vi "ComputerRemote.vi"() -> ()   [LabVIEW 2020]
uses:
  LMH-PS4/Private/Type Defs/Indicators/Controller.ctl
  LMH-PS4/Private/Type Defs/Indicators/Square.ctl
  LMH-PS4/Private/Type Defs/Indicators/X.ctl
  LMH-PS4/Private/Type Defs/Indicators/Circle.ctl
  LMH-PS4/Private/Type Defs/Indicators/Triangle.ctl
  LMH-PS4/Private/Type Defs/Indicators/L1.ctl
  LMH-PS4/Private/Type Defs/Indicators/R1.ctl
  LMH-PS4/Private/Type Defs/Indicators/Share.ctl
  LMH-PS4/Private/Type Defs/Indicators/Options.ctl
  LMH-PS4/Private/Type Defs/Indicators/PS.ctl
  LMH-PS4/Private/Type Defs/Indicators/Pad_Button.ctl
  LMH-PS4/Private/Type Defs/Indicators/Dpad.ctl
  LMH-PS4/Private/Type Defs/Indicators/Slider.ctl
  LMH-PS4/Public/Open First Controller.vi
  LMH-PS4/LMH-PS4.lvlib
  <vilib>/ReMiSYS Technology/RemoteToolkit/Sender/Sender.lvclass
panel:
  out "D-Pad":T1=5
  out "R2":T2 scale=-32768.0..32767.0
  out "L2":T2 scale=-32768.0..32767.0
  in  "IP Address":string="10.12.34.2"
  in  "Stop Button":bool
  out "PS4 Controller":T3={"Square Button"=FALSE, "X Button"=FALSE, "Circle Button"=FALSE, "Triangle Button"=FALSE, "L1"=FALSE, "R1"=FALSE, "Share Button"=FALSE, "Options Button"=FALSE, "PS Button"=FALSE, "Pad Button"=FALSE, "D-Pad"=5, "L2"=0, "R2"=0, "Thumbstick_Left"={[], []}, "Thumbstick_Right"={[], []}} {"R2" scale=-32768.0..32767.0; "L2" scale=-32768.0..32767.0}
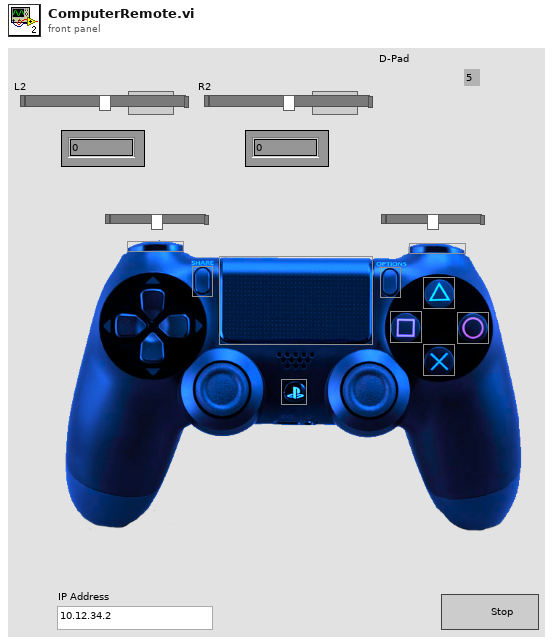
[diagram p1: front panel]
types:
  T1 = typedef "LMH-PS4.lvlib/Dpad.ctl" = u16
  T2 = typedef "LMH-PS4.lvlib/Slider.ctl" = i32
  T3 = typedef "LMH-PS4.lvlib/Controller.ctl" = cluster{"Square Button":T4, "X Button":T5, "Circle Button":T6, "Triangle Button":T7, "L1":T8, "R1":T9, "Share Button":T10, "Options Button":T11, "PS Button":T12, "Pad Button":T13, "D-Pad":T1, "L2":T2, "R2":T2, "Thumbstick_Left":cluster{i32[], i32[]}, "Thumbstick_Right":cluster{i32[], i32[]}}
  T4 = typedef "LMH-PS4.lvlib/Square.ctl" = bool
  T5 = typedef "LMH-PS4.lvlib/X.ctl" = bool
  T6 = typedef "LMH-PS4.lvlib/Circle.ctl" = bool
  T7 = typedef "LMH-PS4.lvlib/Triangle.ctl" = bool
  T8 = typedef "LMH-PS4.lvlib/L1.ctl" = bool
  T9 = typedef "LMH-PS4.lvlib/R1.ctl" = bool
  T10 = typedef "LMH-PS4.lvlib/Share.ctl" = bool
  T11 = typedef "LMH-PS4.lvlib/Options.ctl" = bool
  T12 = typedef "LMH-PS4.lvlib/PS.ctl" = bool
  T13 = typedef "LMH-PS4.lvlib/Pad_Button.ctl" = bool
  T14 = typedef "LMH-PS4.lvlib/PS4 Controller Ref.ctl" = cluster{"Controller Ref":refnum<k1>, "PS4 Events Ref":refnum<event-registration>, "Worker Ref":refnum<vi>}
  T15 = typedef "LMH-PS4.lvlib/Axis.ctl" = cluster{"Left Thumbstick":cluster{"X Axis":i32, "Y Axis":i32}, "Right Thumbstick":cluster{"X Axis":i32, "Y Axis":i32}, "L2":i32, "R2":i32, "D-Pad":T16}
  T16 = typedef "LMH-PS4.lvlib/DPad Enum.ctl" = enum16{"Idle", "Up", "Up / Right", "Right", "Down / Right", "Down", "Down / Left", "Left", "Up / Left"}
  T17 = typedef "LMH-PS4.lvlib/Buttons.ctl" = cluster{"Square":bool, "X":bool, "Circle":bool, "Triangle":bool, "L1":bool, "R1":bool, "L2":bool, "R2":bool, "Share":bool, "Options":bool, "Left Thumbstick":bool, "Right Thumbstick":bool, "Playstation Button":bool, "Pad":bool}
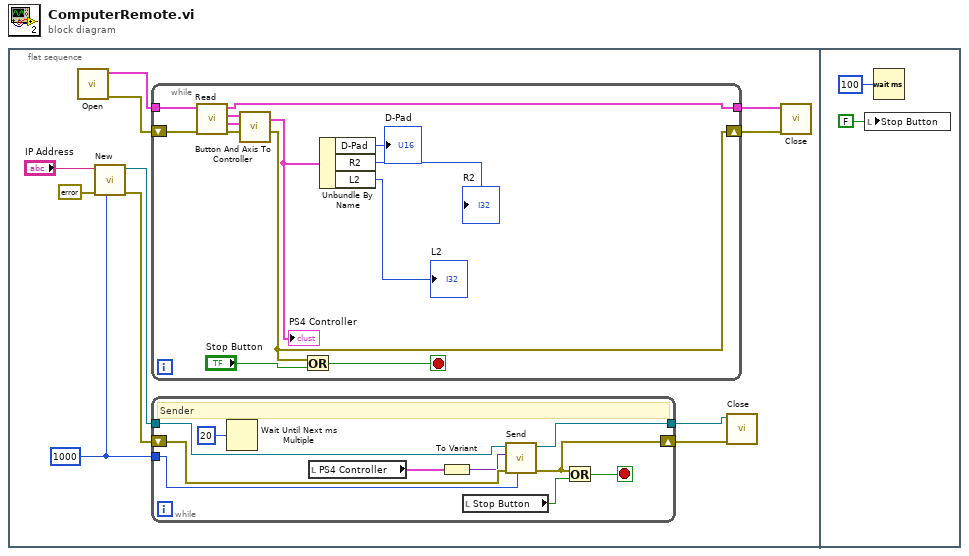
[diagram p0: block diagram]
diagram:
  n1 = flat-sequence {
    frame #0 {
      w5 = 1000 ("Timeout ms (25000)")
      n2 = call-poly "Open.vi"() -> ("Error Out"=w9:errorcluster, "PS4 Controller Ref"=w8:T14)  [unwired: 9 in, 1 out]
      n3 = call <vilib>:"New.vi"("Timeout ms (25000)"=w5, "Error In"=errorcluster {"status"=FALSE, "code"=0, "source"=""}, "IP Address"="IP Address") -> ("Error Out"=w6:errorcluster, "Sender Ref."=w3:refnum<class "Sender.lvclass">)  [unwired: 7 in]
      n4 = while {
        shift-right: [w29] -> w11
        shift-left: w9 -> [w26]
        tunnel: [w28] -> w10
        tunnel: w8 -> [w27]
        stop <- w31 stop-if-true
        n5 = call "Read.vi"("Error In"=w26, "PS4 Controller Ref"=w27) -> ("Error Out"=w29:errorcluster, "All Axis"=w33:T15, "Buttons"=w32:T17, "PS4 Controller Ref"=w28:T14)  [unwired: 6 in]
        n6 = call "Button And Axis To Controller.vi"("All Axis"=w33, "Buttons"=w32) -> ("PS4 Controller"=w25:T3)  [unwired: 5 in]
        "PS4 Controller" <- w25
        n7 = Or(x=w29, y="Stop Button") -> (x .or. y?=w31:bool)
        n8 = Unbundle By Name(w25) -> ("D-Pad"=→"D-Pad":T1, "R2"=→"R2":T2, "L2"=→"L2":T2)
      }
      n9 = while {
        shift-right: [w17] -> w2
        shift-left: w6 -> [w19]
        tunnel: w3 -> [w20]
        tunnel: w5 -> [w15]
        tunnel: [w18] -> w1
        stop <- w21 stop-if-true
        # "Sender"
        n10 = Wait Until Next ms Multiple(millisecond multiple=u32 20) -> ()  [unwired: 1 out]
        n11 = local read "PS4 Controller"() -> (w13:T3)
        n12 = To Variant(anything=w13) -> (Variant=w16:variant)
        n13 = local read "Stop Button"() -> (w12:bool)
        n14 = call <vilib>:"Send.vi"("Timeout ms (1000)"=w15, "Error In"=w19, "Value"=w16, "Sender Ref."=w20) -> ("Error Out"=w17:errorcluster, "Sender Ref."=w18:refnum<class "Sender.lvclass">)  [unwired: 6 in]
        n15 = Or(x=w17, y=w12) -> (x .or. y?=w21:bool)
      }
      n16 = call <vilib>:"Close.vi"("Error In"=w2, "Receiver Ref."=w1) -> ()  [unwired: 9 in, 1 out]
      n17 = call <vilib>:"Close.vi"("Error In"=w11, "PS4 Controller Ref"=w10) -> ()  [unwired: 9 in, 1 out]
    }
    frame #1 {
      n18 = local write "Stop Button"(FALSE ("Stop Button")) -> ()
      n19 = Wait (ms)(milliseconds to wait=u32 100) -> ()  [unwired: 1 out]
    }
  }
